vi "CameraVision_Demo_v01.vi"() -> (4 "图像时间戳":u32=16532020 format="%_32g")   [LabVIEW 2015]
uses:
  MVCAMSDK.dll
  <vilib>/Analysis/NI_AALBase.lvlib
panel:
  out "variance":dbl caption="方差" format="%0.2f"
  out "相机图像":T1(plugin-control)
  out "光强图":u8[](graph)
  in  "自定义分辨率设置":bool
  in  "ROI分辨率":T2
  in  "预设分辨率设置":bool
  in  "预设分辨率":T3(radio)
  out "帧速":u32
  out "帧间耗时\n单位：（0.1ms）":u32
  in  "相机枚举":T4(ring)
  in  "自动曝光模式":bool=TRUE caption="软触发"
  in  "手动曝光模式":bool caption="软触发"
  in  "曝光时间，单位微秒":dbl=11000.0 format="%#_6f"
  in  "硬触发模式":bool caption="软触发"
  in  "软触发模式":bool caption="软触发"
  in  "连续模式":bool caption="软触发"
  in  "软触发一帧":bool caption="软触发"
  in  "读取自定义数据":bool
  out "从相机中读出的字符串(32字节)":string
  in  "写入自定义数据":bool
  in  "要写入相机的字符串(32字节)":string
  in  "拍照":bool
  in  "相机参数":bool=TRUE
  in  "Stop":bool
  in  "激活预览":bool=TRUE
  out "Image":T1(plugin-control)
  # "写入自定义数据"
  # "相机原生分辨率设置"
  # "触发设置"
  # "曝光设置"
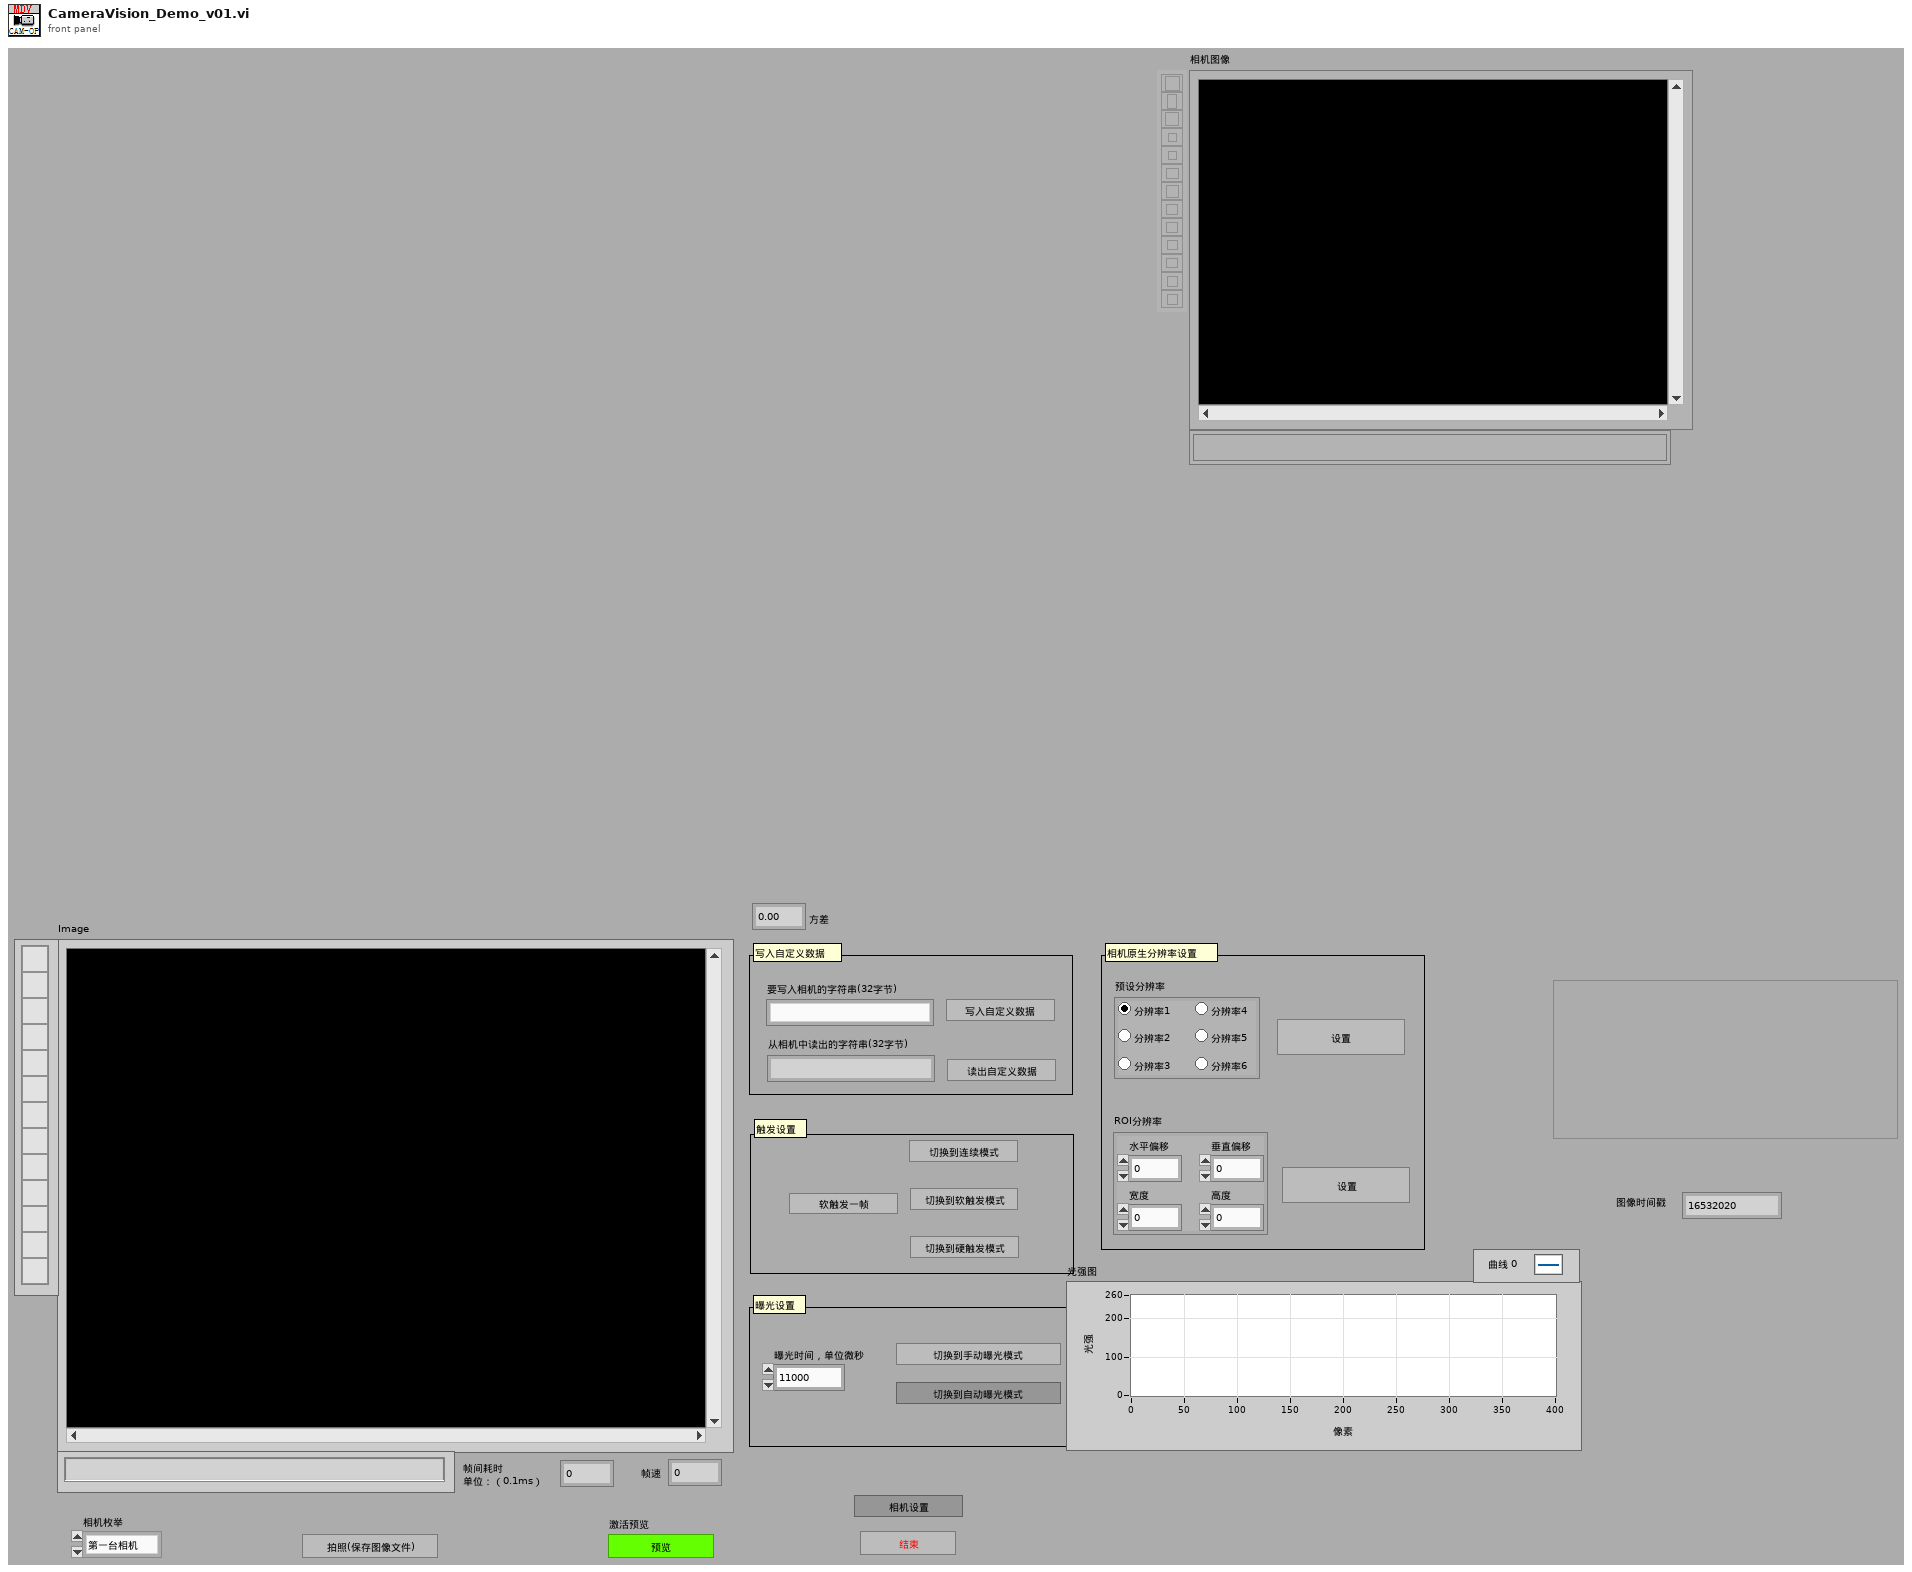
[diagram p1: front panel]
types:
  T1 = typedef "IMAQ Image.ctl" = refnum<image>
  T2 = cluster{"水平偏移":dbl, "垂直偏移":dbl, "宽度":dbl, "高度":dbl}
  T3 = enum32{"分辨率1", "分辨率2", "分辨率3", "分辨率4", "分辨率5", "分辨率6"}
  T4 = enum16{"第一台相机", "第二台相机", "第三台相机", "第四台相机", "第五台相机"}
  T5 = typedef "Image Type" = u32
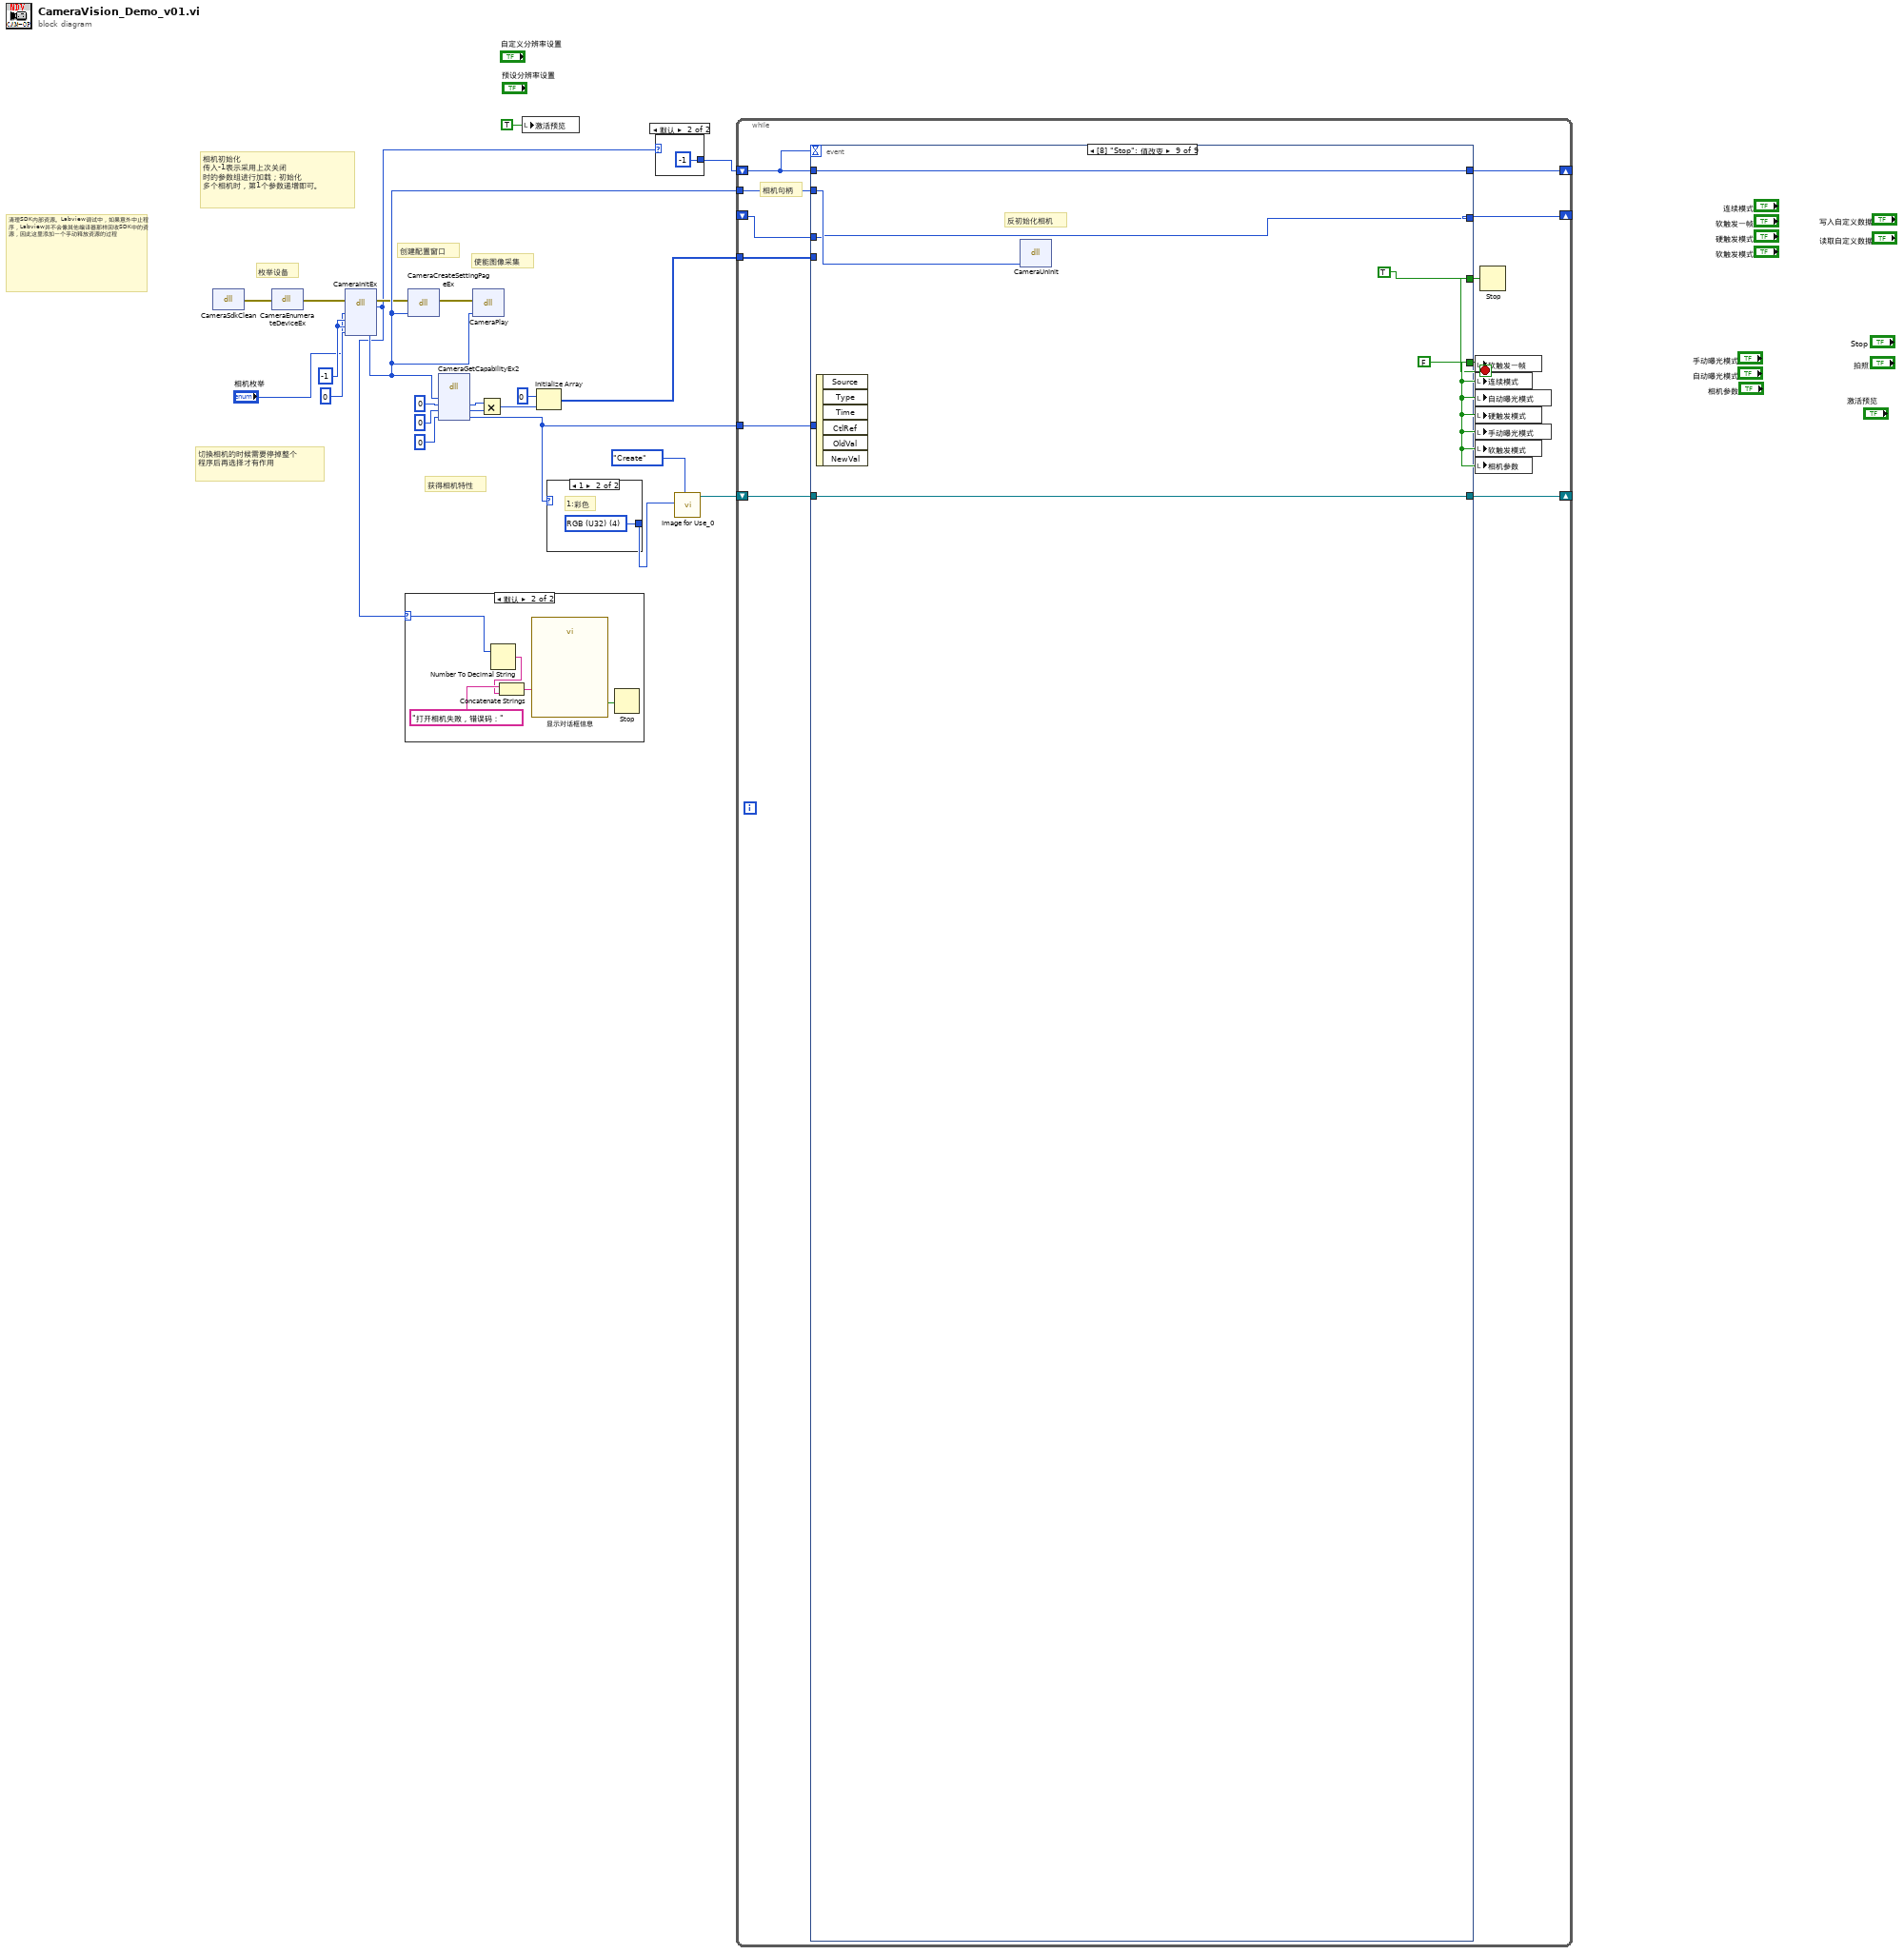
[diagram p0: block diagram]
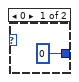
[diagram p2: hidden frame]
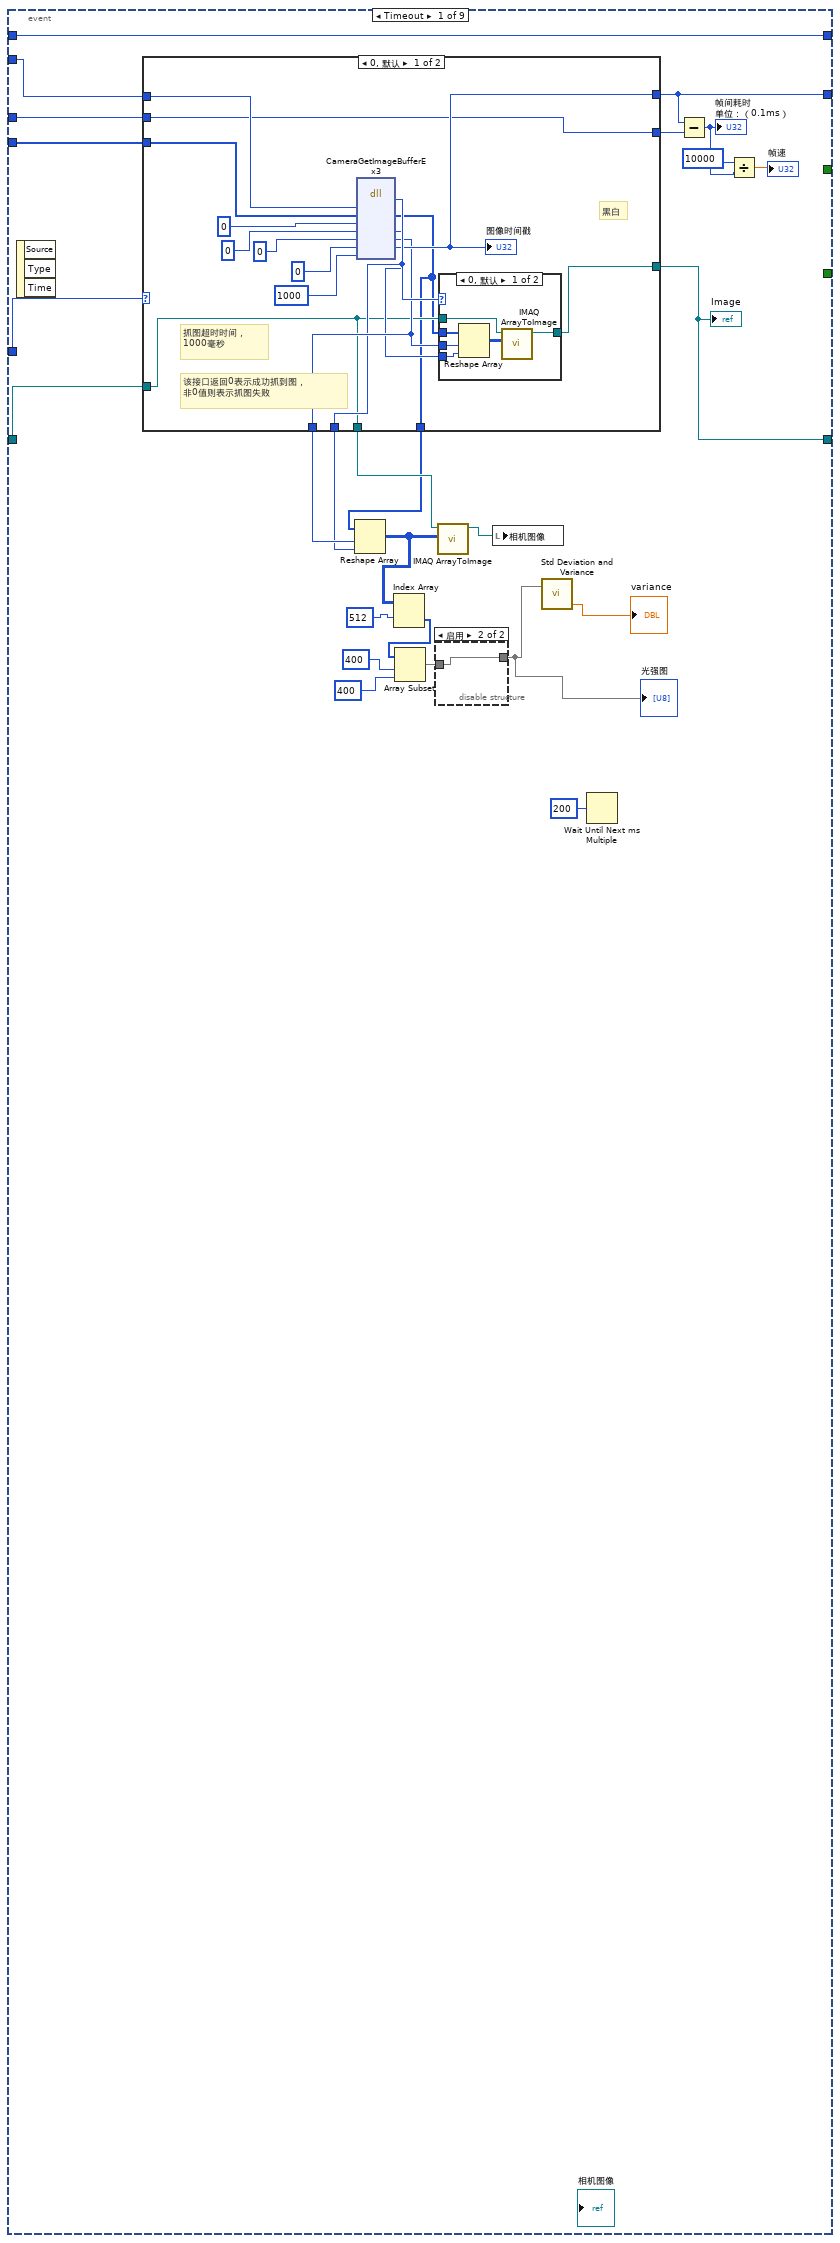
[diagram p4: hidden frame]
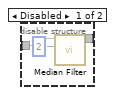
[diagram p5: hidden frame]
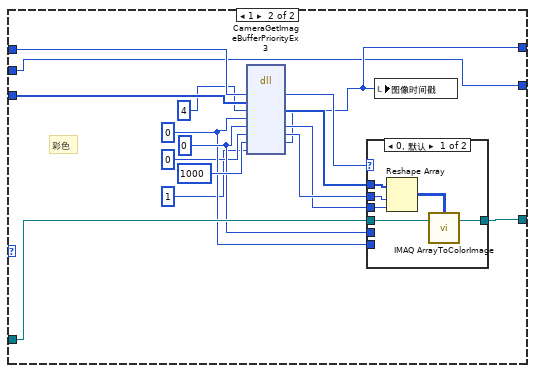
[diagram p7: hidden frame]
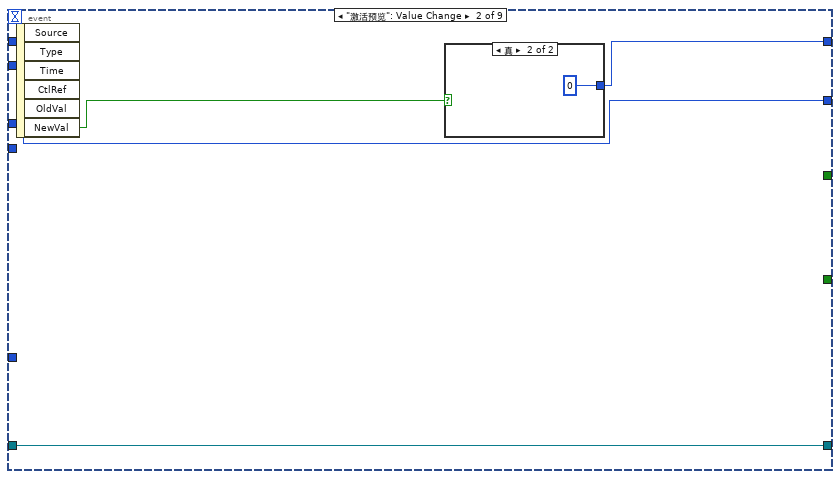
[diagram p9: hidden frame]
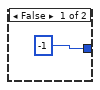
[diagram p10: hidden frame]
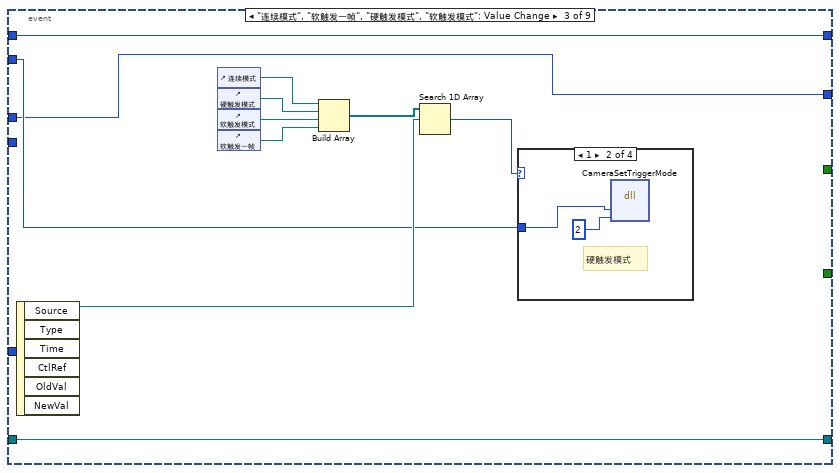
[diagram p11: hidden frame]
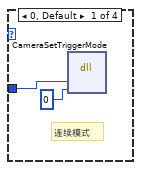
[diagram p12: hidden frame]
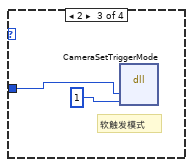
[diagram p13: hidden frame]
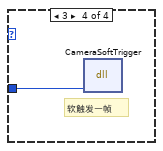
[diagram p14: hidden frame]
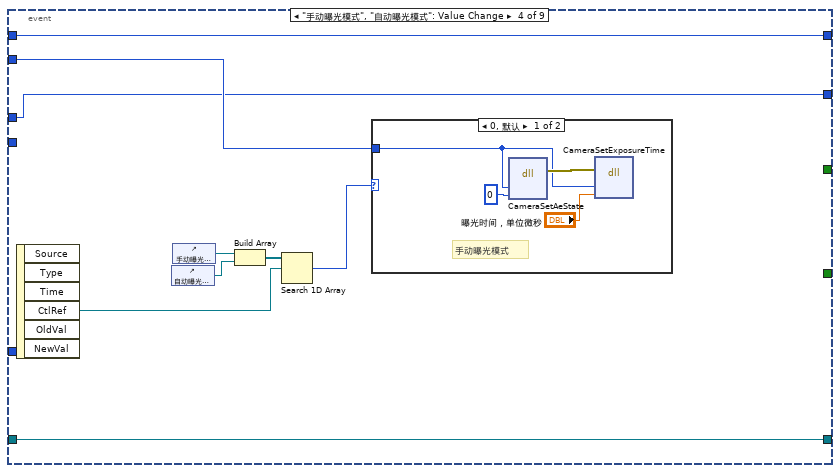
[diagram p15: hidden frame]
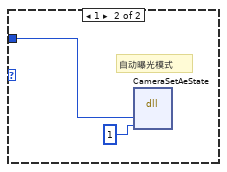
[diagram p16: hidden frame]
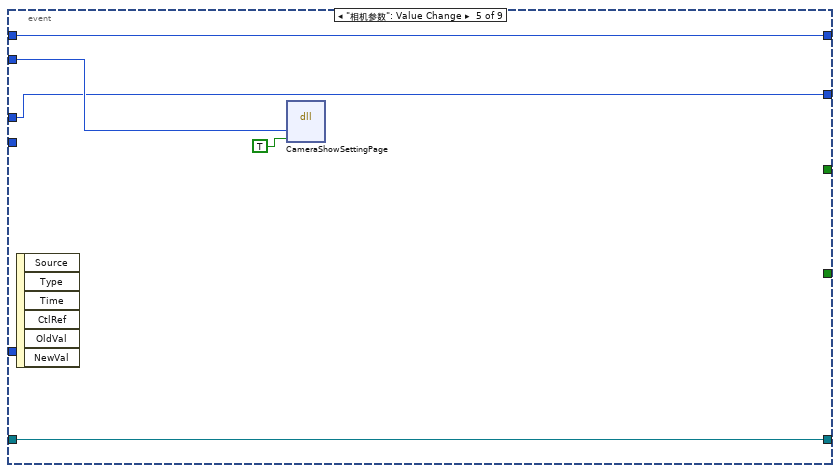
[diagram p17: hidden frame]
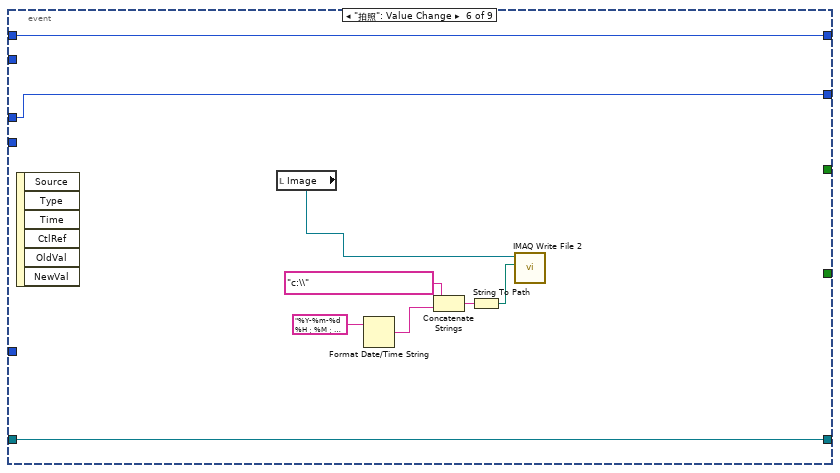
[diagram p18: hidden frame]
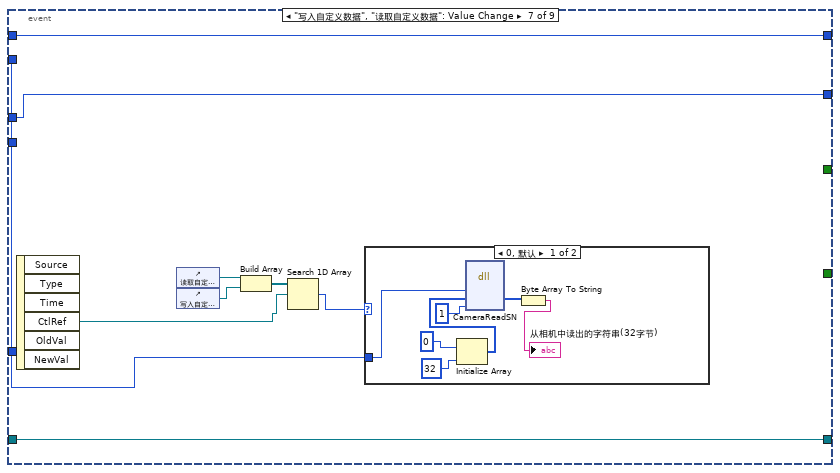
[diagram p19: hidden frame]
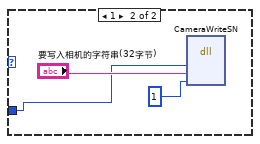
[diagram p20: hidden frame]
diagram:
  w20 = -1
  # "切换相机的时候需要停掉整个\n程序后再选择才有作用"
  # "清理SDK内部资源。Labview调试中，如果意外中止程序，Labview并不会像其他编译器那样回收SDK中的资源，因此这里添加一个手动释放资源的过程"
  # "使能图像采集"
  # "获得相机特性"
  # "创建配置窗口"
  # "相机初始化\n传入-1表示采用上次关闭\n时的参数组进行加载；初始化\n多个相机时，第1个参数递增即可。"
  # "枚举设备"
  n1 = dll-call lib="MVCAMSDK.dll" fn="CameraSdkClean"() -> (error out=w21:errorcluster)  [unwired: 4 in, 1 out]
  n2 = dll-call lib="MVCAMSDK.dll" fn="CameraEnumerateDeviceEx"(error in=w21) -> (error out=w18:errorcluster)  [unwired: 3 in, 1 out]
  n3 = dll-call lib="MVCAMSDK.dll" fn="CameraInitEx"(error in=w18, "相机索引值"="相机枚举", "参数加载方式"=w20, "要加载的参数组索引"=w20, "相机句柄"=0) -> (error out=w7:errorcluster, "返回类型"=w2:i32, "相机句柄"=w9:i32)  [unwired: 5 in, 1 out]
  n4 = case shown="默认" w2 {
    selector: w2 -> [_ w27]
    frame 0 {
    }
    frame Default {
      n5 = Number To Decimal String(number=w27) -> (decimal integer string=w24:string)  [unwired: 1 in]
      n6 = Concatenate Strings("打开相机失败，错误码：" ("字符串"), w24) -> (w26:string)
      n7 = call "显示对话框信息"("Message"=w26) -> ("结束"=w28:bool)  [unwired: 9 in, 1 out]
      n8 = Stop(stop? (T)=w28) -> ()
    }
  }
  n9 = dll-call lib="MVCAMSDK.dll" fn="CameraCreateSettingPageEx"(error in=w7, "相机句柄"=w9) -> (error out=w10:errorcluster)  [unwired: 4 in, 1 out]
  n10 = dll-call lib="MVCAMSDK.dll" fn="CameraGetCapabilityEx2"("相机句柄"=w9, "图像最大宽度"=0, "图像最大高度"=0, "是否是彩色相机(返回0:黑白;1:彩色)"=0) -> ("图像最大宽度"=w12:i32, "图像最大高度"=w11:i32, "是否是彩色相机(返回0:黑白;1:彩色)"=w6:i32)  [unwired: 5 in, 2 out]
  n11 = dll-call lib="MVCAMSDK.dll" fn="CameraPlay"(error in=w10, "相机句柄"=w9) -> ()  [unwired: 4 in, 2 out]
  n12 = Multiply(x=w12, y=w11) -> (x*y=w16:i32)
  n13 = local write "激活预览"(TRUE ("激活预览")) -> ()
  n14 = Initialize Array(0, w16) -> (w8:i32[])
  n15 = case shown="1" w6 {
    tunnel: [_ w29] -> w22
    frame 0, Default {
      # "0:黑白;"
    }
    frame 1 {
      w29 = T5 4 items=["Grayscale (U8)", "Grayscale (I16)", "Grayscale (SGL)", "Complex (CSG)", "RGB (U32)", "HSL (U32)", "RGB (U64)", "Grayscale (U16)"] ("Image Type")
      # "1:彩色"
    }
  }
  n16 = case shown="默认" w2 {
    tunnel: [0 -1] -> w1
    frame 0 {
    }
    frame Default {
    }
  }
  n17 = call "Image for Use_0.vi"("Command"=enum16{"Create", "Use", "Copy in", "Dispose"}."Create", "Image Type"=w22) -> ("Image out"=w5:T1)  [unwired: 8 in, 1 out]
  n18 = while {
    tunnel: w9 -> [w39]
    tunnel: w8 -> [w41]
    tunnel: w6 -> [w42]
    shift-right: [w38] -> _
    shift-left: w1 -> [w37]
    shift-right: [w35] -> _
    shift-left: w5 -> [w40]
    shift-right: [w34] -> _
    shift-left: _ -> [w33]
    stop <- w32 stop-if-true
    # "相机句柄"
    n19 = event shown="[8] \"Stop\": 值改变" {
      selector: _ -> [_ _ _ _ _ _ _ _ _]
      dyn-events: _ -> [_ _ _ _ _ _ _ _ _]
      timeout: w37 -> [_ _ _ _ _ _ _ _ _]
      tunnel: [_ _ _ _ _ _ _ _ TRUE] -> w32
      tunnel: w41 -> [w67 _ _ _ _ _ _ _ _]
      tunnel: w42 -> [w66 _ _ _ _ _ _ _ _]
      tunnel: w39 -> [w68 _ w126 w144 w159 _ w173 w196 w276]
      tunnel: w40 -> [w65 w119 w125 w143 w158 w163 w172 w198 w274]
      tunnel: [w64 w120 w127 w145 w160 w164 w174 w199 w277] -> w38
      tunnel: w37 -> [w64 _ w127 w145 w160 w164 w174 w199 w277]
      tunnel: [_ _ _ _ _ _ _ _ FALSE] -> w36
      tunnel: [w63 w119 w125 w143 w158 w163 w172 w198 w274] -> w35
      tunnel: [w60 w118 w124 w142 w157 w162 w171 w190 w273] -> w34
      tunnel: w33 -> [w62 w118 w124 w142 w157 w162 w171 w190 w273]
      event Timeout {
        n20 = event-data() -> ()  [unwired: 1 in, 3 out]
        n21 = case shown="0, 默认" w66 {
          tunnel: w67 -> [w87 w110]
          tunnel: w65 -> [w74 w109]
          tunnel: w68 -> [w79 w108]
          tunnel: [w80 w98] -> w63
          tunnel: [w78 w97] -> w60
          tunnel: w62 -> [w77 w96]
          tunnel: [w77 w96] -> w61
          tunnel: [w76 _] -> w48
          tunnel: [w75 _] -> w47
          tunnel: [w74 _] -> w46
          tunnel: [w73 _] -> w45
          frame 0, Default {
            # "黑白"
            # "该接口返回0表示成功抓到图，\n非0值则表示抓图失败"
            # "抓图超时时间，\n1000毫秒"
            n22 = dll-call lib="MVCAMSDK.dll" fn="CameraGetImageBufferEx3"("相机句柄"=w79, "图像数据缓冲区"=w87, "图像输出格式(0:8位灰度;1:24位彩色;2:32位彩色，3：BGR24彩色 4：BGRA32位彩色)"=0, "图像宽度"=0, "图像高度"=0, "时间戳(单位为100微秒)"=0, "抓图超时时间(毫秒)"=1000) -> ("返回类型"=w82:i32, "图像数据缓冲区"=w73:u8[], "图像宽度"=w75:i32, "图像高度"=w76:i32, "时间戳(单位为100微秒)"=w78:u32)  [unwired: 6 in, 2 out]
            "图像时间戳" <- w78
            n23 = case shown="0, 默认" w82 {
              tunnel: w73 -> [w93 _]
              tunnel: w74 -> [w90 w94]
              tunnel: w76 -> [w92 _]
              tunnel: w75 -> [w91 _]
              tunnel: [w88 w94] -> w80
              frame 0, Default {
                n24 = Reshape Array(w93, w92, w91) -> (w89:u8[][])
                n25 = call "IMAQ ArrayToImage"("Image Pixels (U8)"=w89, "Image"=w90) -> ("Image Out"=w88:T1)  [unwired: 8 in, 1 out]
              }
              frame -12 {
              }
            }
          }
          frame 1 {
            w100 = 0
            w101 = 0
            # "彩色"
            n26 = dll-call lib="MVCAMSDK.dll" fn="CameraGetImageBufferPriorityEx3"("相机句柄"=w108, "图像数据缓冲区"=w110, "图像输出格式(0:8位灰度;1:24位彩色;2:32位彩色)"=4, "图像宽度"=w100, "图像高度"=w101, "时间戳（单位为100微秒）"=0, "抓图超时时间(毫秒)"=1000, "取图优先级(0: 取最旧   1:取最新)"=1) -> ("返回类型"=w102:i32, "图像数据缓冲区"=w105:u32[], "图像宽度"=w103:i32, "图像高度"=w104:i32, "时间戳（单位为100微秒）"=w97:u32)  [unwired: 7 in, 2 out]
            n27 = case shown="0, 默认" w102 {
              tunnel: w105 -> [w115 _]
              tunnel: w109 -> [w114 w117]
              tunnel: w104 -> [w113 _]
              tunnel: w103 -> [w112 _]
              tunnel: w101 -> [_ _]
              tunnel: w100 -> [_ _]
              tunnel: [w111 w117] -> w98
              frame 0, Default {
                n28 = Reshape Array(w115, w113, w112) -> (w116:u32[][])
                n29 = call "IMAQ ArrayToColorImage"("Image Pixels (U32)"=w116, "Image"=w114) -> ("Image Out"=w111:T1)  [unwired: 3 in, 1 out]
              }
              frame -12 {
              }
            }
            n30 = local write "图像时间戳"(w97) -> ()
          }
        }
        "Image" <- w63
        n31 = Reshape Array(w45, w48, w47) -> (w44:u8[][])
        n32 = Index Array(array=w44, index (row)=512 ("索引 (行)")) -> (element=w51:u8[])  [unwired: 1 in]
        n33 = Array Subset(array=w51, index=400 ("索引"), length=400 ("长度")) -> (w53:u8[])
        n34 = disable-structure shown="启用" {
          disable-tunnel: w53 -> [w71 w72]
          disable-tunnel: [w69 w72] -> w56
          frame Disabled {
            n35 = call <vilib>:"Median Filter.vi"("left rank"=2, "X"=w71) -> ("Filtered X"=w69:dbl[])  [unwired: 8 in, 1 out]
          }
          frame Enabled {
          }
        }
        "光强图" <- w56
        n36 = call "IMAQ ArrayToImage"("Image Pixels (U8)"=w44, "Image"=w46) -> ("Image Out"=w49:T1)  [unwired: 8 in, 1 out]
        n37 = local write "相机图像"(w49) -> ()
        n38 = call <vilib>:"Std Deviation and Variance.vi"("X"=w56) -> ("variance"=→"variance":dbl)  [unwired: 1 in, 2 out]
        n39 = Wait Until Next ms Multiple(millisecond multiple=u32 200 ("毫秒倍数")) -> ()  [unwired: 1 out]
        n40 = Subtract(x=w60, y=w61) -> (x-y=w59:u32)
        "帧间耗时\n单位：（0.1ms）" <- w59
        n41 = Divide(x=u32 10000 ("帧间耗时"), y=w59) -> (x/y=→"帧速":dbl)
      }
      event "激活预览": Value Change {
        n42 = event-data() -> ("NewVal"=w121:bool)  [unwired: 1 in, 5 out]
        n43 = case shown="真" w121 {
          tunnel: [-1 0] -> w120
          frame False {
          }
          frame True {
          }
        }
      }
      event "连续模式", "软触发一帧", "硬触发模式", "软触发模式": Value Change {
        n44 = event-data() -> ("CtlRef"=w129:refnum<vi>)  [unwired: 1 in, 5 out]
        n45 = control-ref of="连续模式"() -> (w131:refnum<vi>)
        n46 = control-ref of="硬触发模式"() -> (w132:refnum<vi>)
        n47 = control-ref of="软触发模式"() -> (w133:refnum<vi>)
        n48 = control-ref of="软触发一帧"() -> (w134:refnum<vi>)
        n49 = Build Array ("创建数组")(w131, w132, w133, w134) -> (w130:refnum<vi>[])
        n50 = Search 1D Array(1D array=w130, element=w129) -> (index of element=w128:i32)  [unwired: 1 in]
        n51 = case shown="1" w128 {
          tunnel: w126 -> [w135 w137 w139 w141]
          frame 0, Default {
            # "连续模式"
            n52 = dll-call lib="MVCAMSDK.dll" fn="CameraSetTriggerMode"("相机句柄"=w135, "模式"=0) -> ()  [unwired: 6 in, 2 out]
          }
          frame 1 {
            # "硬触发模式"
            n53 = dll-call lib="MVCAMSDK.dll" fn="CameraSetTriggerMode"("相机句柄"=w137, "模式"=2) -> ()  [unwired: 6 in, 2 out]
          }
          frame 2 {
            # "软触发模式"
            n54 = dll-call lib="MVCAMSDK.dll" fn="CameraSetTriggerMode"("相机句柄"=w139, "模式"=1) -> ()  [unwired: 6 in, 2 out]
          }
          frame 3 {
            # "软触发一帧"
            n55 = dll-call lib="MVCAMSDK.dll" fn="CameraSoftTrigger"("相机句柄"=w141) -> ()  [unwired: 5 in, 2 out]
          }
        }
      }
      event "手动曝光模式", "自动曝光模式": Value Change {
        n56 = event-data() -> ("CtlRef"=w148:refnum<vi>)  [unwired: 1 in, 5 out]
        n57 = control-ref of="自动曝光模式"() -> (w146:refnum<vi>)
        n58 = control-ref of="手动曝光模式"() -> (w149:refnum<vi>)
        n59 = Build Array ("创建数组")(w149, w146) -> (w150:refnum<vi>[])
        n60 = Search 1D Array(1D array=w150, element=w148) -> (index of element=w147:i32)  [unwired: 1 in]
        n61 = case shown="0, 默认" w147 {
          tunnel: w144 -> [w151 w155]
          frame 0, Default {
            # "手动曝光模式"
            n62 = dll-call lib="MVCAMSDK.dll" fn="CameraSetAeState"("相机句柄"=w151, "曝光模式(0手动，1自动)"=0) -> (error out=w154:errorcluster)  [unwired: 6 in, 1 out]
            n63 = dll-call lib="MVCAMSDK.dll" fn="CameraSetExposureTime"(error in=w154, "相机句柄"=w151, "曝光时间，单位微秒"="曝光时间，单位微秒") -> ()  [unwired: 5 in, 2 out]
          }
          frame 1 {
            # "自动曝光模式"
            n64 = dll-call lib="MVCAMSDK.dll" fn="CameraSetAeState"("相机句柄"=w155, "曝光模式(0手动，1自动)"=1) -> ()  [unwired: 6 in, 2 out]
          }
        }
      }
      event "相机参数": Value Change {
        n65 = event-data() -> ()  [unwired: 1 in, 6 out]
        n66 = dll-call lib="MVCAMSDK.dll" fn="CameraShowSettingPage"("相机句柄"=w159, "状态"=TRUE) -> ()  [unwired: 6 in, 2 out]
      }
      event "拍照": Value Change {
        n67 = event-data() -> ()  [unwired: 1 in, 6 out]
        n68 = local read "Image"() -> (w165:T1)
        n69 = Format Date/Time String(time format string (%c)="%Y-%m-%d %H：%M：%S.bmp ") -> (date/time string=w169:string)  [unwired: 2 in]
        n70 = Concatenate Strings("c:\\", w169) -> (w166:string)
        n71 = String To Path(string=w166) -> (path=w168:path)
        n72 = call-poly "IMAQ Write File 2"("File Path"=w168, "Image"=w165) -> ()  [unwired: 8 in, 2 out]
      }
      event "写入自定义数据", "读取自定义数据": Value Change {
        n73 = event-data() -> ("CtlRef"=w176:refnum<vi>)  [unwired: 1 in, 5 out]
        n74 = control-ref of="读取自定义数据"() -> (w178:refnum<vi>)
        n75 = control-ref of="写入自定义数据"() -> (w177:refnum<vi>)
        n76 = Build Array ("创建数组")(w178, w177) -> (w179:refnum<vi>[])
        n77 = Search 1D Array(1D array=w179, element=w176) -> (index of element=w175:i32)  [unwired: 1 in]
        n78 = case shown="0, 默认" w175 {
          tunnel: w173 -> [w180 w187]
          frame 0, Default {
            n79 = Initialize Array(0, 32) -> (w184:i32[])
            n80 = dll-call lib="MVCAMSDK.dll" fn="CameraReadSN"("相机句柄"=w180, "序列号"=w184, "序列号级别，[0,1,2],0级为只读，1,2级可写"=1) -> ("序列号"=w182:u8[])  [unwired: 6 in, 2 out]
            n81 = Byte Array To String(unsigned byte array=w182) -> (string=→"从相机中读出的字符串(32字节)":string)
          }
          frame 1 {
            n82 = dll-call lib="MVCAMSDK.dll" fn="CameraWriteSN"("相机句柄"=w187, "序列号(固定为32个字节)"="要写入相机的字符串(32字节)", "序列号级别，[0,1,2]对应3级序列号，其中0级为只读，1,2级可写"=1) -> ()  [unwired: 7 in, 2 out]
          }
        }
      }
      event "预设分辨率设置", "自定义分辨率设置": Value Change {
        n83 = event-data() -> ("CtlRef"=w192:refnum<vi>)  [unwired: 1 in, 5 out]
        n84 = control-ref of="预设分辨率设置"() -> (w194:refnum<vi>)
        n85 = control-ref of="自定义分辨率设置"() -> (w193:refnum<vi>)
        n86 = Build Array ("创建数组")(w194, w193) -> (w195:refnum<vi>[])
        n87 = Search 1D Array(1D array=w195, element=w192) -> (index of element=w191:i32)  [unwired: 1 in]
        n88 = case shown="1" w191 {
          tunnel: "预设分辨率" -> [w201 _]
          tunnel: w196 -> [w200 w262]
          frame 0, Default {
            n89 = case shown="\"分辨率2\"" w201 {
              tunnel: w200 -> [w202 w221 w222 w232 w242 w252]
              frame "分辨率1", Default {
                n90 = dll-call lib="MVCAMSDK.dll" fn="CameraSetImageResolutionEx"("相机句柄"=w202, "预设分辨率索引"=0, "Mode"=0, "ModeSize"=u32 0, "x"=0, "y"=u32 0 ("ModeSize"), "width"=0, "height"=0, "ZoomWidth"=0, "ZoomHeight"=0) -> ()  [unwired: 14 in, 2 out]
              }
              frame "分辨率2" {
                n91 = dll-call lib="MVCAMSDK.dll" fn="CameraSetImageResolutionEx"("相机句柄"=w221, "预设分辨率索引"=1, "Mode"=0, "ModeSize"=u32 0, "x"=0, "y"=u32 0 ("ModeSize"), "width"=0, "height"=0, "ZoomWidth"=0, "ZoomHeight"=0) -> ()  [unwired: 14 in, 2 out]
              }
              frame "分辨率3" {
                n92 = dll-call lib="MVCAMSDK.dll" fn="CameraSetImageResolutionEx"("相机句柄"=w222, "预设分辨率索引"=2, "Mode"=0, "ModeSize"=u32 0, "x"=0, "y"=u32 0 ("ModeSize"), "width"=0, "height"=0, "ZoomWidth"=0, "ZoomHeight"=0) -> ()  [unwired: 14 in, 2 out]
              }
              frame "分辨率4" {
                n93 = dll-call lib="MVCAMSDK.dll" fn="CameraSetImageResolutionEx"("相机句柄"=w232, "预设分辨率索引"=3, "Mode"=0, "ModeSize"=u32 0, "x"=0, "y"=u32 0 ("ModeSize"), "width"=0, "height"=0, "ZoomWidth"=0, "ZoomHeight"=0) -> ()  [unwired: 14 in, 2 out]
              }
              frame "分辨率5" {
                n94 = dll-call lib="MVCAMSDK.dll" fn="CameraSetImageResolutionEx"("相机句柄"=w242, "预设分辨率索引"=4, "Mode"=0, "ModeSize"=u32 0, "x"=0, "y"=u32 0 ("ModeSize"), "width"=0, "height"=0, "ZoomWidth"=0, "ZoomHeight"=0) -> ()  [unwired: 14 in, 2 out]
              }
              frame "分辨率6" {
                n95 = dll-call lib="MVCAMSDK.dll" fn="CameraSetImageResolutionEx"("相机句柄"=w252, "预设分辨率索引"=5, "Mode"=0, "ModeSize"=u32 0, "x"=0, "y"=u32 0 ("ModeSize"), "width"=0, "height"=0, "ZoomWidth"=0, "ZoomHeight"=0) -> ()  [unwired: 14 in, 2 out]
              }
            }
          }
          frame 1 {
            n96 = Unbundle("ROI分辨率") -> ("水平偏移"=w264:dbl, "垂直偏移"=w265:dbl, "宽度"=w266:dbl, "高度"=w267:dbl)
            n97 = dll-call lib="MVCAMSDK.dll" fn="CameraSetImageResolutionEx"("相机句柄"=w262, "预设分辨率索引"=255, "Mode"=0, "ModeSize"=u32 0, "x"=w264, "y"=w265, "width"=w266, "height"=w267, "ZoomWidth"=0, "ZoomHeight"=u32 0 ("ModeSize")) -> ()  [unwired: 14 in, 2 out]
          }
        }
      }
      event "Stop": Value Change {
        # "反初始化相机"
        n98 = event-data() -> ()  [unwired: 1 in, 6 out]
        n99 = dll-call lib="MVCAMSDK.dll" fn="CameraUnInit"("相机句柄"=w276) -> ()  [unwired: 5 in, 2 out]
      }
    }
    n100 = local write "软触发一帧"(w36) -> ()
    n101 = local write "连续模式"(w36) -> ()
    n102 = local write "自动曝光模式"(w36) -> ()
    n103 = local write "硬触发模式"(w36) -> ()
    n104 = local write "手动曝光模式"(w36) -> ()
    n105 = local write "软触发模式"(w36) -> ()
    n106 = local write "相机参数"(w36) -> ()
    n107 = Stop(stop? (T)=w32) -> ()
  }
